vi "Filter Words.vi"(11 "Array in":string[](array[string])) -> (3 "Array out":string[](array[string]))   [LabVIEW 2021, in "Text-Based VI Icon.lvlib"]
uses:
  Text-Based VI Icon.lvlib
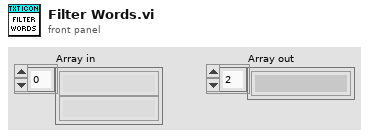
[diagram p1: front panel]
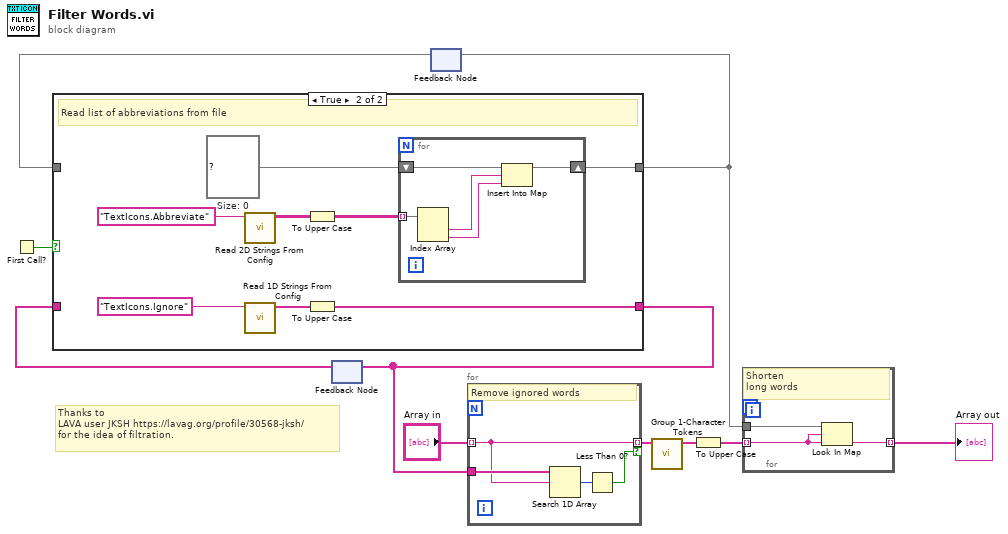
[diagram p0: block diagram]
diagram:
  # "Thanks to\nLAVA user JKSH https://lavag.org/profile/30568-jksh/\nfor the idea of filtration."
  n1 = First Call?() -> (First Call?: T/F=w5:bool)
  n2 = feedback #1() -> (w7:string[])  [unwired: 1 in]
  n3 = feedback #2() -> (w4:map{string, string})  [unwired: 1 in]
  n4 = case shown="True" w5 {
    tunnel: [w12 w18] -> w6
    tunnel: w4 -> [w12 _]
    tunnel: [w11 w13] -> w8
    tunnel: w7 -> [w11 _]
    frame False {
    }
    frame True {
      w19 = map{string, string} {}  # Size: 0
      # "Read list of abbreviations from file"
      n5 = call "Read 2D Strings From Config.vi"("key"="TextIcons.Abbreviate" ("section")) -> ("2D array strings"=w17:string[][])  [unwired: 10 in]
      n6 = call "Read 1D Strings From Config.vi"("key"="TextIcons.Ignore" ("section")) -> ("1D array strings"=w14:string[])  [unwired: 10 in]
      n7 = To Upper Case(1:w17) -> (0:w16:string[][])
      n8 = To Upper Case(1:w14) -> (0:w13:string[])
      n9 = for {
        tunnel: w16 -> [w23] mode=indexing
        shift-right: [w24] -> w18
        shift-left: w19 -> [w25]
        n10 = Index Array(array=w23) -> (element #1=w22:string, element #2=w21:string)  [unwired: 2 in]
        n11 = Insert Into Map(map in=w25, key=w22, value=w21) -> (map out=w24:map{string, string})  [unwired: 2 out]
      }
    }
  }
  n12 = feedback-in #1(w8) -> ()
  n13 = feedback-in #2(w6) -> ()
  n14 = for {
    tunnel: "Array in" -> [w28] mode=indexing
    tunnel: [w28] -> w9 mode=indexing if=w26
    tunnel: w8 -> [w29]
    # "Remove ignored words"
    n15 = Search 1D Array(1D array=w29, element=w28) -> (index of element=w27:i32)  [unwired: 1 in]
    n16 = Less Than 0?(x=w27) -> (x < 0?=w26:bool)
  }
  n17 = call "Group 1-Character Tokens.vi"("Array"=w9) -> ("Grouped Tokens"=w2:string[])  [unwired: 10 in]
  n18 = To Upper Case(1:w2) -> (0:w1:string[])
  n19 = for {
    tunnel: w1 -> [w31] mode=indexing
    tunnel: [w30] -> w3 mode=indexing
    tunnel: w6 -> [w32]
    # "Shorten\nlong words"
    n20 = Look In Map(map=w32, key=w31, default value=w31) -> (value=w30:string)  [unwired: 1 out]
  }
  "Array out" <- w3
